vi "Read IP.vi"(8 "error in (no error)":errorcluster, 11 "gRPC Container in":refnum<class "XNET.CAN.BusMonitor.API.lvclass">) -> (0 "error out":errorcluster, 2 "IP":string, 3 "gRPC Container out":refnum<class "XNET.CAN.BusMonitor.API.lvclass">)   [LabVIEW 2025, in "XNET.CAN.BusMonitor.API.lvlib" / "XNET.CAN.BusMonitor.API.lvclass"]
uses:
  XNET.CAN.BusMonitor.API.lvclass
  XNET.CAN.BusMonitor.API.lvclass/XNET.CAN.BusMonitor.API.ctl
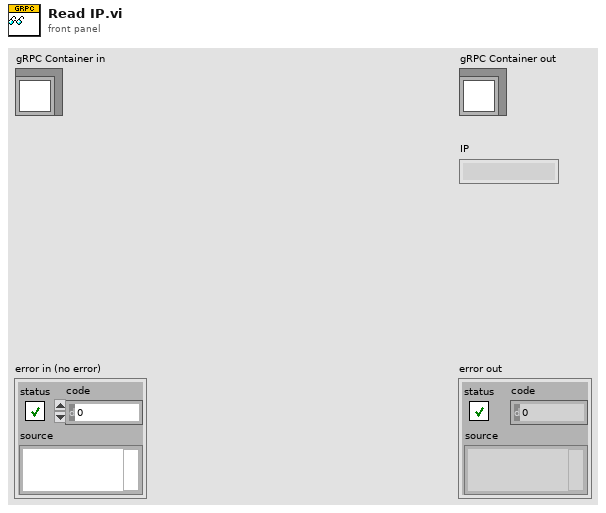
[diagram p1: front panel]
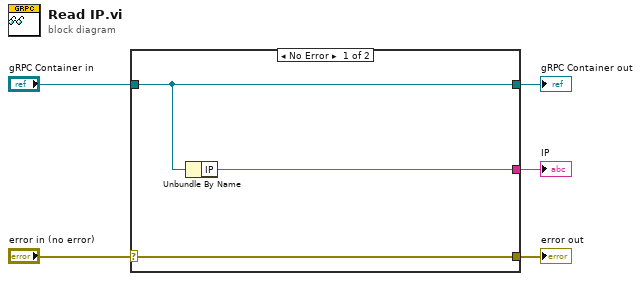
[diagram p0: block diagram]
diagram:
  n1 = case shown="No Error" "error in (no error)" {
    selector: "error in (no error)" -> [w8 w9]
    tunnel: [w8 w9] -> w4
    tunnel: [w7 w10] -> w2
    tunnel: "gRPC Container in" -> [w7 w10]
    tunnel: [w6 _] -> w1
    frame No Error {
      n2 = Unbundle By Name(w7) -> ("IP"=w6:string)
    }
    frame Error {
    }
  }
  "error out" <- w4
  "gRPC Container out" <- w2
  "IP" <- w1
